vi "Headless Video Analyzer.vi"() -> ()   [LabVIEW 2018]
uses:
  Shared/Roughness Parameters STYP.ctl
  Classes/Message/Message.lvclass
  Private/Headless Video Analyzer Status STYP.ctl
  Classes/Video File/Video File.lvclass
  Classes/Video Frame/Video Frame.lvclass
  <vilib>/vision/Image Controls.llb/IMAQ Image.ctl
  <userlib>/Jet Engineering/JET_QSM/Code/Private/JET_QSM_InvalidOption STYP.ctl
  Classes/Video File/Video File.lvclass/Video File.ctl
  <userlib>/Jet Engineering/JET_QSM/Code/Private/JET_QSM - Add State [String API].vi
  905395b3-fc2a-4912-8404-34f757d12cd7.vi
  Classes/Video File/Read Number of Frames.vi
  Classes/Video File/Read Frame Number.vi
  Datalogger/Messages/Datalogger Headers Set Message/Datalogger Headers Set Message.lvclass
  C:/Users/aaron.jencks/Documents/GitHub/emerson_seed_object_detection/LabVIEW/Projects/Paul's Video Viewer/Classes/Message/Message.lvclass
  Datalogger/Messages/Datalogger Data Save Message.lvclass
  Classes/STOP Message/STOP.lvclass
  Classes/Depth Data Message/Depth Data Message.lvclass
  <vilib>/Utility/error.llb/Trim Whitespace.vi
  <vilib>/Utility/error.llb/Error Cluster From Error Code.vi
panel:
  out "Frame Number":u32
  out "Progress":dbl(slide) scale=0.0..100.0
  out "Depth":T1(plugin-control)
  out "Ready?":bool
  in  "stop":bool
  out "File Opened?":bool
  out "Frame Count":u32
  out "Roughness Parameters":T2
  in  "Path":path
  out "RGB":T1(plugin-control)
  out "Recent states before Error (with tick counts) 2":string="0.167 sec ago: VI Initialize\n0.167 sec ago: Window Open\n0.110 sec ago: Control Update\n0.110 sec ago: Indicator Update\n0.000 sec ago: Error Handler\r\n"
  out "error out":errorcluster
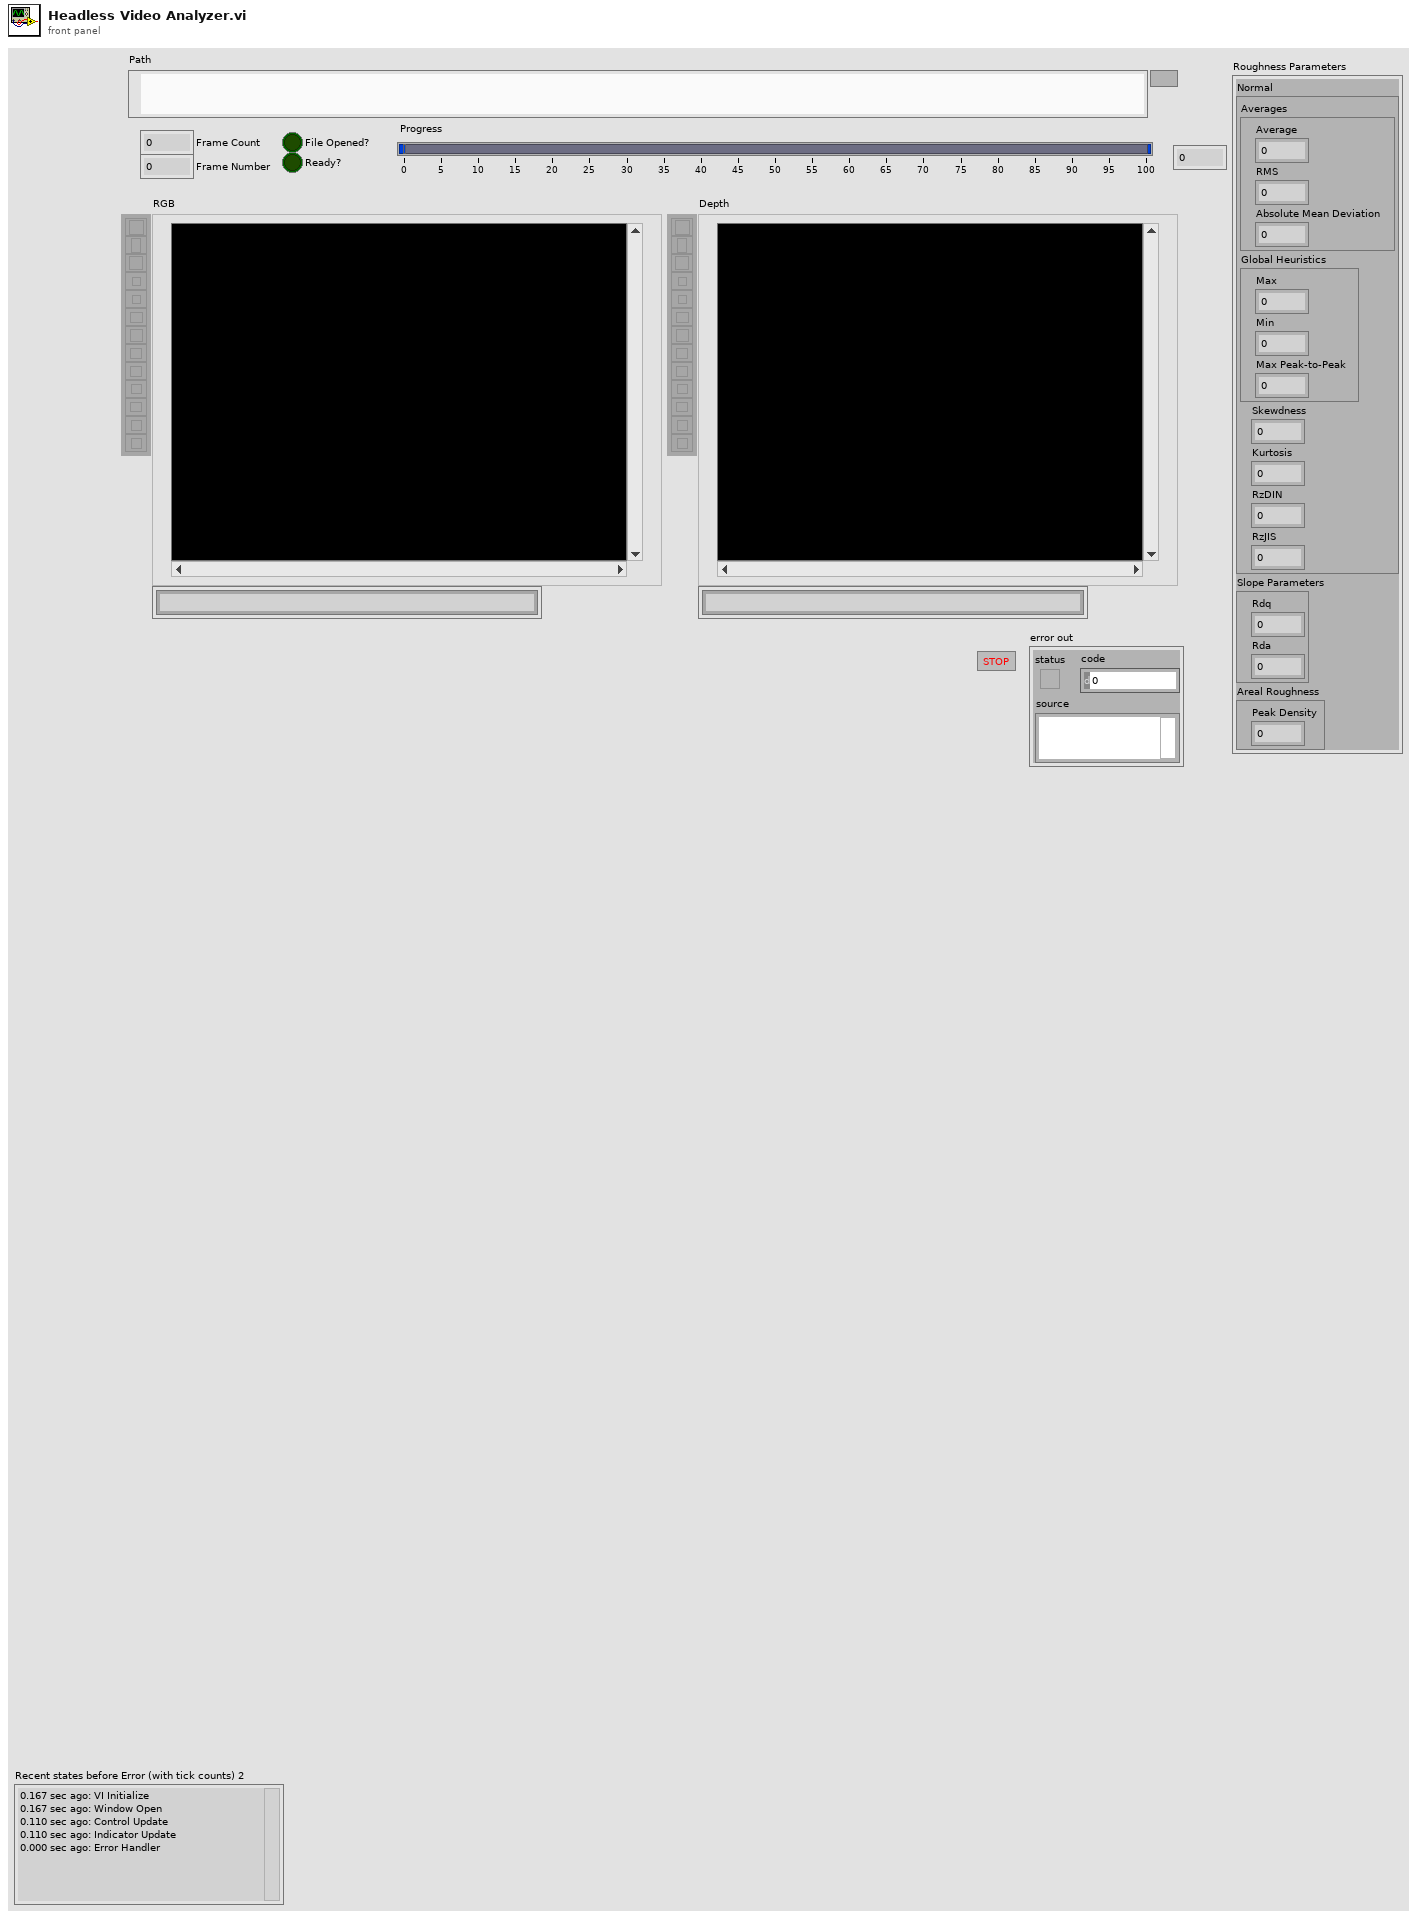
[diagram p1: front panel]
types:
  T1 = typedef "IMAQ Image.ctl" = refnum<image>
  T2 = typedef "Roughness Parameters STYP.ctl" = cluster{"Normal":cluster{"Averages":cluster{"Average":dbl, "RMS":dbl, "Absolute Mean Deviation":dbl}, "Global Heuristics":cluster{"Max":dbl, "Min":dbl, "Max Peak-to-Peak":dbl}, "Skewdness":dbl, "Kurtosis":dbl, "RzDIN":dbl, "RzJIS":dbl}, "Slope Parameters":cluster{"Rdq":dbl, "Rda":dbl}, "Areal Roughness":cluster{"Peak Density":dbl}}
  T3 = typedef "Headless Video Analyzer Status STYP.ctl" = cluster{"VI":cluster{"error":errorcluster, "isExiting?":bool}, "UserLoggedIn?":bool, "data log queue":refnum<queue>, "stop queue":refnum<queue>, "ready queue":refnum<queue>, "Files":cluster{"Depth File":refnum<class "Video File.lvclass">, "RGB File":refnum<class "Video File.lvclass">}, "Frames":cluster{"Depth Frame":refnum<class "Video Frame.lvclass">, "RGB Frame":refnum<class "Video Frame.lvclass">}, "Images":cluster{"Depth Placeholder":T1, "RGB Placeholder":T1}, "Playing?":bool, "Processed Frame":T2}
  T4 = typedef "JET_QSM_InvalidOption STYP.ctl" = enum16{"Ignore", "Dialog", "Error"}
  T5 = typedef "JET_QSM_Refnum STYP.ctl" = cluster{"state":cluster{"queue":refnum<queue>, "idle":string, "error":string, "STOP":string}, "debug":cluster{"enabled?":bool, "queue":refnum<queue>}, "Invalid.option":T4, "QSM.Name":string}
  T6 = enum32{"invalid app kind", "Development System", "Run Time System", "Student Edition", "Embedded LabVIEW", "Evaluation", "Custom"}
  T7 = typedef "JET_QSM_Element STYP.ctl" = cluster{"state":string, "data":variant, "comment":string}
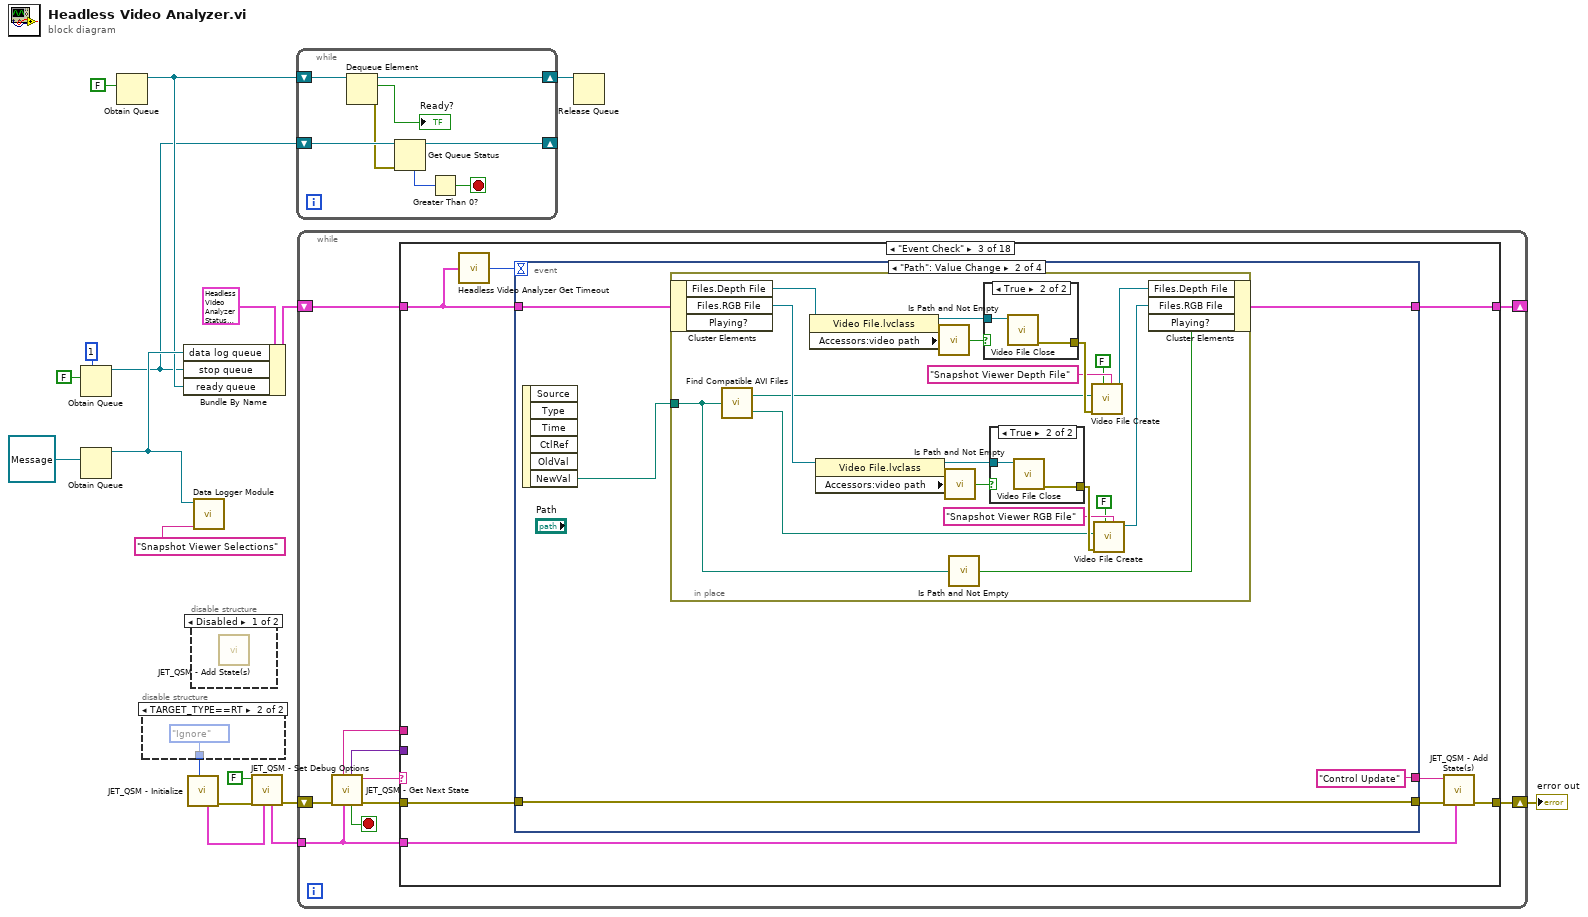
[diagram p0: block diagram]
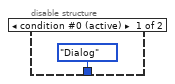
[diagram p2: hidden frame]
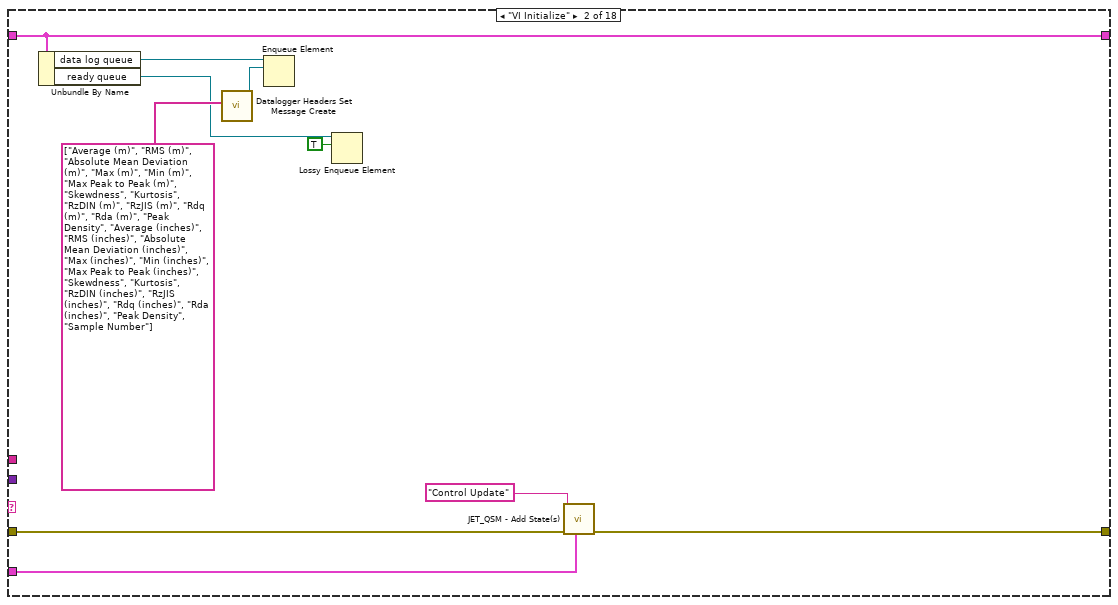
[diagram p5: hidden frame]
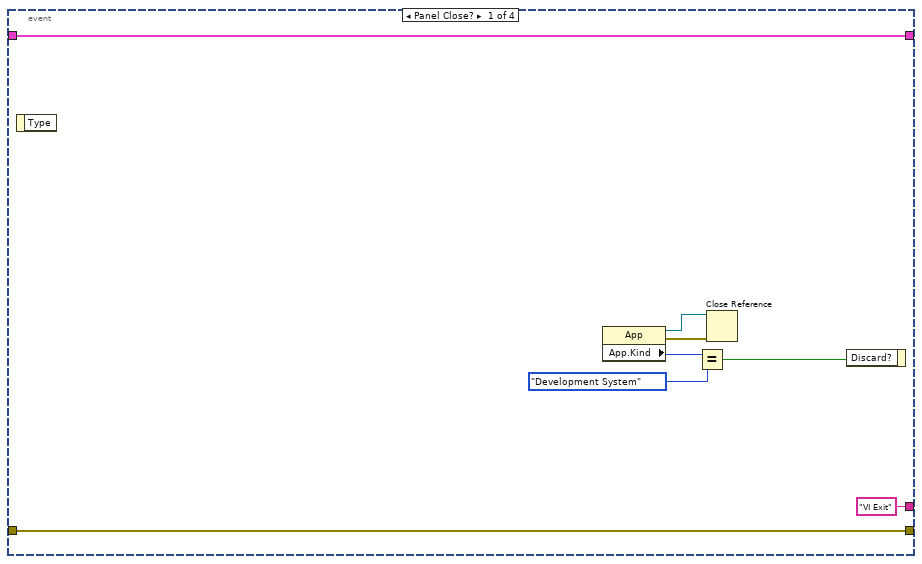
[diagram p6: hidden frame]
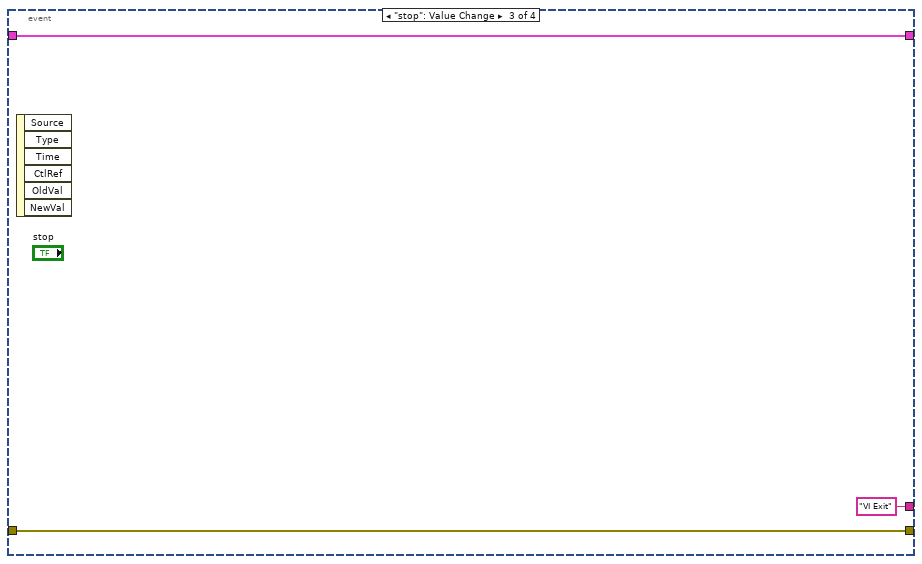
[diagram p9: hidden frame]
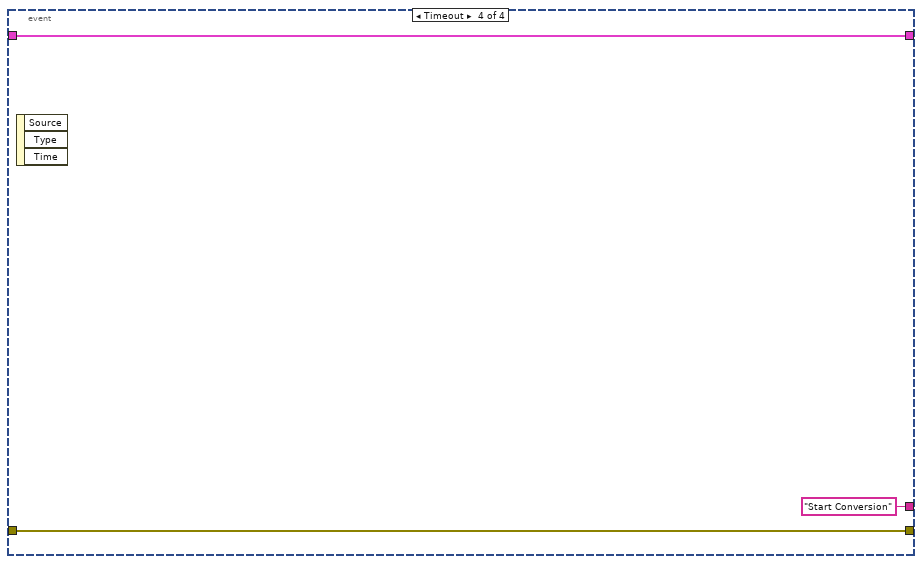
[diagram p10: hidden frame]
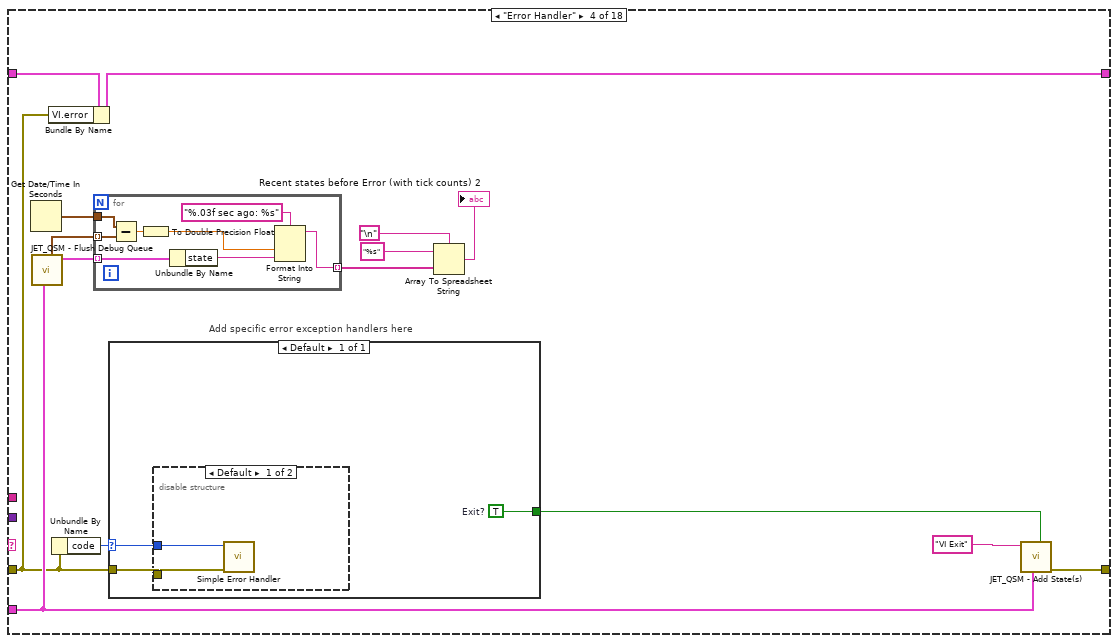
[diagram p11: hidden frame]
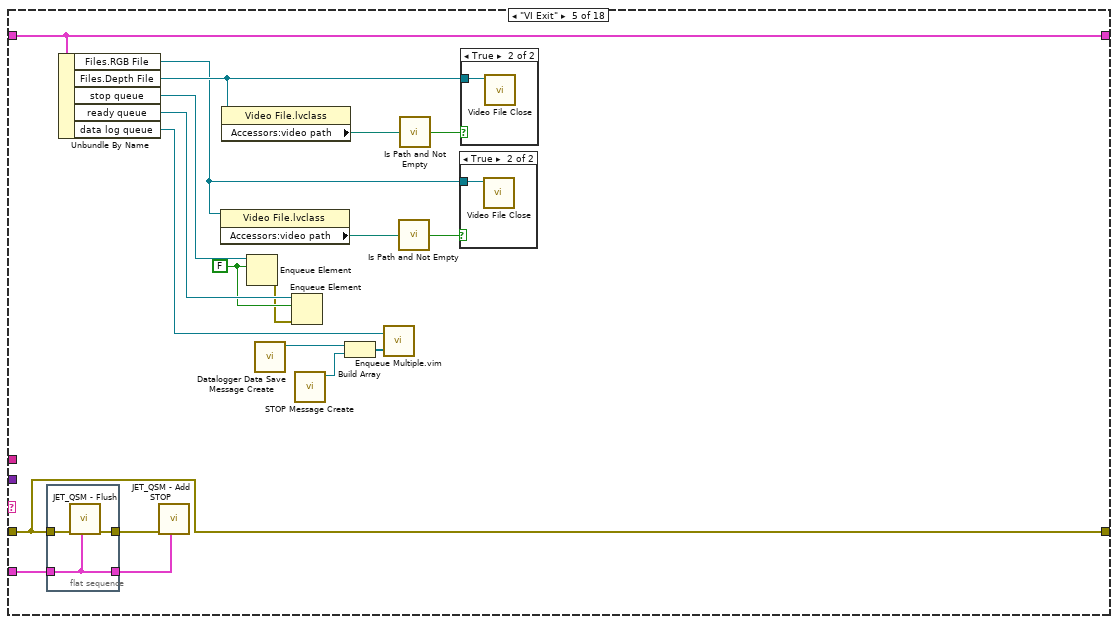
[diagram p13: hidden frame]
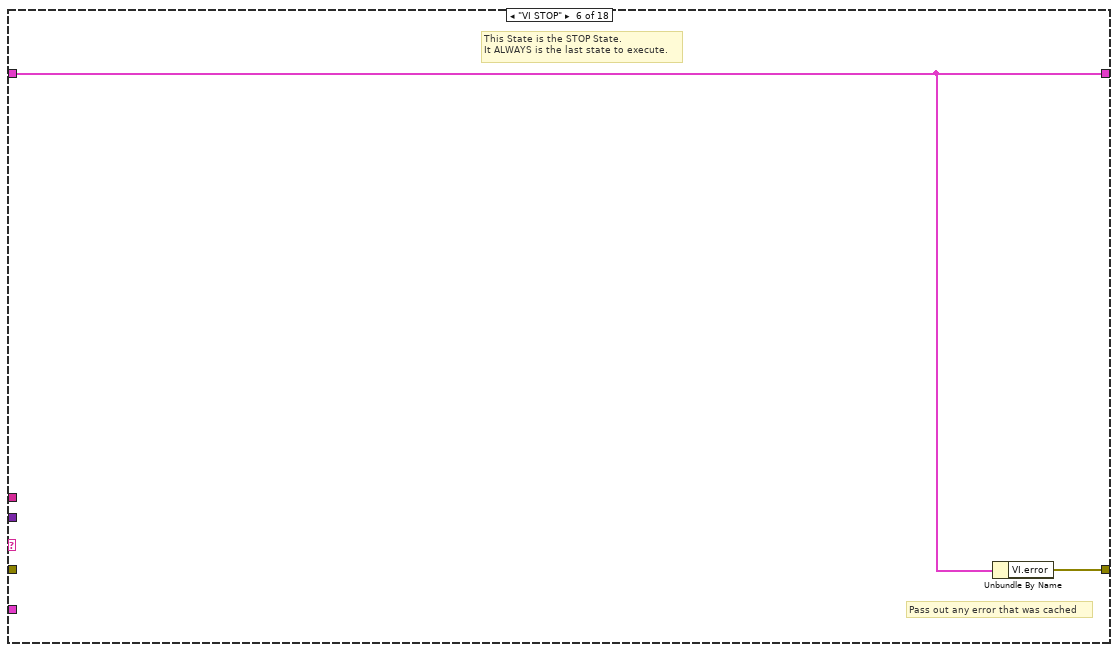
[diagram p16: hidden frame]
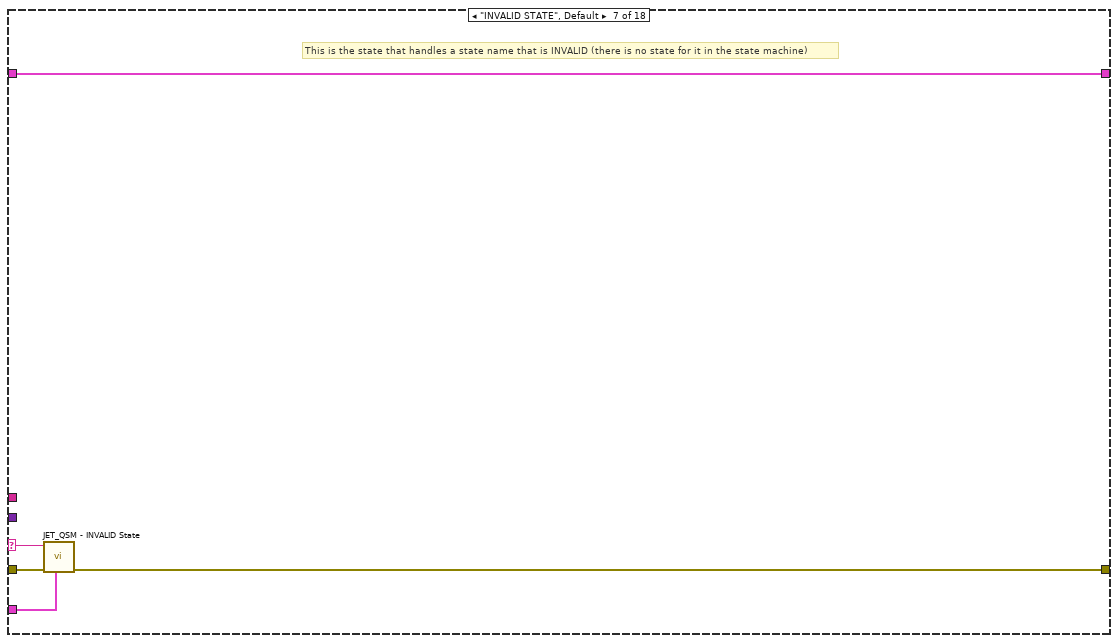
[diagram p17: hidden frame]
diagram:
  n1 = Obtain Queue(max queue size (-1, unlimited)=1, element data type=FALSE) -> (queue out=w4:refnum<queue>)  [unwired: 3 in, 2 out]
  n2 = Obtain Queue(element data type=refnum<class "Message.lvclass"> refnum ("Message.lvclass")) -> (queue out=w8:refnum<queue>)  [unwired: 4 in, 2 out]
  n3 = Obtain Queue(element data type=FALSE) -> (queue out=w5:refnum<queue>)  [unwired: 4 in, 2 out]
  n4 = disable-structure shown="TARGET_TYPE==RT" {
    disable-tunnel: [JET_QSM_InvalidOption_STYP."Dialog" ("invalid state action (Dialog)") JET_QSM_InvalidOption_STYP."Ignore" ("invalid state action (Dialog)")] -> w18
    frame condition #0 (active) {
    }
    frame condition #1 {
    }
  }
  n5 = Bundle By Name(cluster=T3 {"VI"={"error"={"status"=FALSE, "code"=0, "source"=""}, "isExiting?"=FALSE}, "UserLoggedIn?"=FALSE, "data log queue"=refnum, "stop queue"=refnum, "ready queue"=refnum, "Files"={"Depth File"=refnum, "RGB File"=refnum}, "Frames"={"Depth Frame"=refnum, "RGB Frame"=refnum}, "Images"={"Depth Placeholder"=refnum, "RGB Placeholder"=refnum}, "Playing?"=FALSE, "Processed Frame"={"Normal"={"Averages"={"Average"=0.0, "RMS"=0.0, "Absolute Mean Deviation"=0.0}, "Global Heuristics"={"Max"=0.0, "Min"=0.0, "Max Peak-to-Peak"=0.0}, "Skewdness"=0.0, "Kurtosis"=0.0, "RzDIN"=0.0, "RzJIS"=0.0}, "Slope Parameters"={"Rdq"=0.0, "Rda"=0.0}, "Areal Roughness"={"Peak Density"=0.0}}} ("Status"), "data log queue"=w8, "stop queue"=w4, "ready queue"=w5) -> (w9:T3)
  n6 = call <userlib>:"JET_QSM - Initialize.vi"("invalid state action (Dialog)"=w18) -> ("error out"=w12:errorcluster, "Jet_QSM refnum"=w15:T5)  [unwired: 9 in]
  n7 = disable-structure shown="Disabled" {
    frame Disabled {
      n8 = call-poly <userlib>:"JET_QSM - Add State(s).vi"() -> ()  [unwired: 11 in, 1 out]
    }
    frame Enabled {
    }
  }
  n9 = call "Data Logger Module.vi"("Identifier"="Snapshot Viewer Selections", "Message queue"=w8) -> ()  [unwired: 10 in]
  n10 = call <userlib>:"JET_QSM - Set Debug Options.vi"("Jet_QSM refnum"=w15, "error in (no error)"=w12, "debug.enabled? (F)"=FALSE) -> ("error out"=w13:errorcluster, "Jet_QSM ref"=w14:T5)  [unwired: 7 in]
  n11 = while {
    shift-right: [w26] -> w3
    shift-left: w5 -> [w28]
    shift-right: [w22] -> _
    shift-left: w4 -> [w25]
    stop <- w23 stop-if-true
    n12 = Dequeue Element(queue=w28) -> (queue out=w26:refnum<queue>, element=→"Ready?":bool, error out=w21:errorcluster)  [unwired: 2 in, 1 out]
    n13 = Get Queue Status(queue=w25, error in (no error)=w21) -> (queue out=w22:refnum<queue>, # elements in queue=w24:i32)  [unwired: 1 in, 6 out]
    n14 = Greater Than 0?(x=w24) -> (x > 0?=w23:bool)
  }
  n15 = while {
    tunnel: w14 -> [w34]
    shift-right: [w32] -> _
    shift-left: w9 -> [w33]
    shift-right: [w31] -> w17
    shift-left: w13 -> [w38]
    stop <- w35 stop-if-true
    n16 = call <userlib>:"JET_QSM - Get Next State.vi"("Jet_QSM refnum"=w34, "error in (no error)"=w38) -> ("error out"=w37:errorcluster, "state"=w36:string, "Stop Loop?"=w35:bool, "state data"=w30:variant, "state comment"=w29:string)  [unwired: 5 in]
    n17 = case shown="\"Event Check\"" w36 {
      selector: w36 -> [_ _ _ _ _ _ w158 _ _ _ _ _ _ _ _ _ _ _]
      tunnel: w37 -> [w39 w49 w58 w103 w148 _ w159 w161 w163 w165 w174 w193 w210 w215 w219 w220 w226 w246]
      tunnel: w34 -> [_ w50 w57 w108 w146 _ w157 _ _ _ w172 _ _ _ _ _ w227 _]
      tunnel: w33 -> [w40 w46 w52 w104 w144 w154 w160 w162 w164 w166 w170 w192 w208 w211 w218 w221 w224 w245]
      tunnel: [w40 w46 w53 w102 w144 w154 w160 w162 w164 w166 w170 w190 w206 w211 w218 w221 w224 w245] -> w32
      tunnel: [w39 w48 w55 w109 w148 w155 w156 w161 w163 w165 w173 w193 w210 w215 w219 w220 w225 w246] -> w31
      tunnel: w30 -> [_ _ _ _ _ _ _ _ _ _ _ _ _ _ _ _ _ _]
      tunnel: w29 -> [_ _ _ _ _ _ _ _ _ _ _ _ _ _ _ _ _ _]
      frame "------ Standard States ------" {
        # "Standard States are required states for a JET_QSM State Machine\n\nTheir names may be changed; use the Initialize function to specify the new names"
        # "This is a section header; the state is never expected to execute"
      }
      frame "VI Initialize" {
        n18 = Unbundle By Name(w46) -> ("data log queue"=w45:refnum<queue>, "ready queue"=w42:refnum<queue>)
        n19 = call "Datalogger Headers Set Message Create.vi"("Headers"=string[] ["Average (m)", "RMS (m)", "Absolute Mean Deviation (m)", "Max (m)", "Min (m)", "Max Peak to Peak (m)", "Skewdness", "Kurtosis", "RzDIN (m)", "RzJIS (m)", "Rdq (m)", "Rda (m)", "Peak Density", "Average (inches)", "RMS (inches)", "Absolute Mean Deviation (inches)", "Max (inches)", "Min (inches)", "Max Peak to Peak (inches)", "Skewdness", "Kurtosis", "RzDIN (inches)", "RzJIS (inches)", "Rdq (inches)", "Rda (inches)", "Peak Density", "Sample Number"]) -> ("Datalogger Headers Set Message out"=w44:refnum<class "Datalogger Headers Set Message.lvclass">)  [unwired: 9 in, 1 out]
        n20 = Enqueue Element(queue=w45, element=w44) -> ()  [unwired: 2 in, 3 out]
        n21 = Lossy Enqueue Element(queue=w42, element=TRUE) -> ()  [unwired: 1 in, 4 out]
        n22 = call-poly <userlib>:"JET_QSM - Add State(s).vi"("Jet_QSM refnum"=w50, "error in (no error)"=w49, "state(s)"="Control Update") -> ("error out"=w48:errorcluster)  [unwired: 8 in]
      }
      frame "Event Check" {
        n23 = call "Headless Video Analyzer Get Timeout.vi"("Status"=w52) -> ("timeout"=w51:i32)
        n24 = event shown="[1] \"Path\": Value Change" {
          selector: _ -> [_ _ _ _]
          dyn-events: _ -> [_ _ _ _]
          timeout: w51 -> [_ _ _ _]
          tunnel: w58 -> [w60 w71 w97 w100]
          tunnel: ["VI Exit" ("state(s)") "Control Update" ("state(s)") "VI Exit" ("state(s)") "Start Conversion" ("state(s)")] -> w56
          tunnel: [w60 w71 w97 w100] -> w54
          tunnel: w52 -> [w59 w69 w98 w101]
          tunnel: [w59 w68 w98 w101] -> w53
          event Panel Close? {
            n25 = event-data() -> ()  [unwired: 1 in, 1 out]
            n26 = property class="App"() -> (reference out=w62:refnum<vi>, error out=w63:errorcluster, "App.Kind"=w66:T6)  [unwired: 2 in]
            n27 = Equal?(x=w66, y=T6."Development System") -> (x = y?=w64:bool)
            n28 = Close Reference(reference=w62, error in (no error)=w63) -> ()  [unwired: 1 out]
            n29 = event-data("Discard?"=w64) -> ()  [unwired: 1 in, 1 out]
          }
          event "Path": Value Change {
            n30 = event-data() -> ("NewVal"=w67:path)  [unwired: 1 in, 5 out]
            n31 = in-place {
              in-place-border: w67 -> [w75]
              n32 = in-place-cluster #1(w69) -> ("Files.Depth File"=w91:refnum<class "Video File.lvclass">, "Files.RGB File"=w84:refnum<class "Video File.lvclass">)  [unwired: 1 out]
              n33 = call "Find Compatible AVI Files.vi"("Video Path"=w75) -> ("RGB Path"=w76:path, "Depth Path"=w77:path)  [unwired: 2 in]
              n34 = property class="Video File.lvclass"(reference=w91) -> (reference out=w88:refnum<class "Video File.lvclass">, "Accessors:video path"=w90:path)  [unwired: 1 in, 1 out]
              n35 = property class="Video File.lvclass"(reference=w84) -> (reference out=w82:refnum<class "Video File.lvclass">, "Accessors:video path"=w83:path)  [unwired: 1 in, 1 out]
              n36 = call <vilib>:"Is Path and Not Empty.vi"("path"=w90) -> ("Is Path and Not Empty?"=w89:bool)  [unwired: 4 in]
              n37 = call <vilib>:"Is Path and Not Empty.vi"("path"=w83) -> ("Is Path and Not Empty?"=w81:bool)  [unwired: 4 in]
              n38 = call <vilib>:"Is Path and Not Empty.vi"("path"=w75) -> ("Is Path and Not Empty?"=w74:bool)  [unwired: 4 in]
              n39 = case shown="True" w89 {
                tunnel: w88 -> [_ w95]
                tunnel: [_ w94] -> w86
                frame False {
                }
                frame True {
                  n40 = call-dynamic "Video File Close.vi"("Video File in"=w95) -> ("error out"=w94:errorcluster)  [unwired: 9 in, 1 out]
                }
              }
              n41 = case shown="True" w81 {
                tunnel: w82 -> [_ w93]
                tunnel: [_ w92] -> w80
                frame False {
                }
                frame True {
                  n42 = call-dynamic "Video File Close.vi"("Video File in"=w93) -> ("error out"=w92:errorcluster)  [unwired: 9 in, 1 out]
                }
              }
              n43 = call "Video File Create.vi"("Identifier"="Snapshot Viewer Depth File", "Loop? (T)"=FALSE, "error in (no error)"=w86, "Video Path (\"\")"=w77) -> ("Video File out"=w87:refnum<class "Video File.lvclass">)  [unwired: 6 in, 1 out]
              n44 = call "Video File Create.vi"("Identifier"="Snapshot Viewer RGB File", "Loop? (T)"=FALSE, "error in (no error)"=w80, "Video Path (\"\")"=w76) -> ("Video File out"=w78:refnum<class "Video File.lvclass">)  [unwired: 6 in, 1 out]
              n45 = in-place-cluster #1("Files.Depth File"=w87, "Files.RGB File"=w78, "Playing?"=w74) -> (w68:T3)
            }
          }
          event "stop": Value Change {
            n46 = event-data() -> ()  [unwired: 1 in, 6 out]
          }
          event Timeout {
            n47 = event-data() -> ()  [unwired: 1 in, 3 out]
          }
        }
        n48 = call-poly <userlib>:"JET_QSM - Add State(s).vi"("Jet_QSM refnum"=w57, "error in (no error)"=w54, "state(s)"=w56) -> ("error out"=w55:errorcluster)  [unwired: 8 in]
      }
      frame "Error Handler" {
        # "Add specific error exception handlers here"
        n49 = Get Date/Time In Seconds() -> (seconds since 1Jan1904=w112:timestamp)
        n50 = call <userlib>:"JET_QSM - Flush Debug Queue.vi"("Jet_QSM refnum"=w108) -> ("QSM Elements"=w110:T7[], "Timestamps"=w111:timestamp[])  [unwired: 8 in, 1 out]
        n51 = Bundle By Name(cluster=w104, "VI.error"=w103) -> (w102:T3)
        n52 = Unbundle By Name(w103) -> ("code"=w105:i32)
        n53 = for {
          tunnel: w110 -> [w124] mode=indexing
          tunnel: [w122] -> w114 mode=indexing
          tunnel: w112 -> [w119]
          tunnel: w111 -> [w120] mode=indexing
          n54 = Subtract(x=w119, y=w120) -> (x-y=w118:dbl)
          n55 = To Double Precision Float(number=w118) -> (double precision float=w117:dbl)
          n56 = Unbundle By Name(w124) -> ("state"=w123:string)
          n57 = Format Into String(format string="%.03f sec ago: %s", w117, w123) -> (resulting string=w122:string)  [unwired: 2 in, 1 out]
        }
        n58 = case shown="Default" w105 {
          selector: w105 -> [w126]
          tunnel: [w127] -> w106
          tunnel: w103 -> [w125]
          frame Default {
            w127 = TRUE  # Exit?
            n59 = disable-structure shown="Default" {
              disable-tunnel: w126 -> [w129 _]
              disable-tunnel: w125 -> [w128 _]
              frame condition #0 (active) {
                n60 = call <vilib>:"Simple Error Handler.vi"("error code (no error:0)"=w129, "error in (no error)"=w128) -> ()  [unwired: 3 in, 5 out]
              }
              frame condition #1 {
              }
            }
          }
        }
        n61 = Array To Spreadsheet String(delimiter (Tab)="\n", array=w114, 3:"%s" ("format string")) -> (spreadsheet string=→"Recent states before Error (with tick counts) 2":string)
        n62 = call-poly <userlib>:"JET_QSM - Add State(s).vi"("act? (T)"=w106, "Jet_QSM refnum"=w108, "state(s)"="VI Exit") -> ("error out"=w109:errorcluster)  [unwired: 8 in]
      }
      frame "VI Exit" {
        w138 = FALSE ("element")
        n63 = flat-sequence {
          tunnel: w148 -> [w153]
          tunnel: [w152] -> w147
          tunnel: w146 -> [w151]
          tunnel: [w151] -> w145
          frame #0 {
            n64 = call <userlib>:"JET_QSM - Flush.vi"("Jet_QSM ref"=w151, "error in (no error)"=w153) -> ("error out"=w152:errorcluster)  [unwired: 8 in, 1 out]
          }
        }
        n65 = Unbundle By Name(w144) -> ("Files.RGB File"=w130:refnum<class "Video File.lvclass">, "Files.Depth File"=w141:refnum<class "Video File.lvclass">, "stop queue"=w140:refnum<queue>, "ready queue"=w139:refnum<queue>, "data log queue"=w134:refnum<queue>)
        n66 = call <userlib>:"JET_QSM - Add STOP.vi"("Jet_QSM refnum"=w145, "error in (no error)"=w147) -> ()  [unwired: 9 in, 1 out]
        n67 = property class="Video File.lvclass"(reference=w130) -> ("Accessors:video path"=w132:path)  [unwired: 1 in, 2 out]
        n68 = property class="Video File.lvclass"(reference=w141) -> ("Accessors:video path"=w143:path)  [unwired: 1 in, 2 out]
        n69 = Enqueue Element(queue=w140, element=w138) -> (error out=w137:errorcluster)  [unwired: 2 in, 2 out]
        n70 = call "Datalogger Data Save Message Create.vi"() -> ("Datalogger Data Save Message out"=w136:refnum<class "Datalogger Data Save Message.lvclass">)  [unwired: 10 in, 1 out]
        n71 = Enqueue Element(queue=w139, element=w138, error in (no error)=w137) -> ()  [unwired: 1 in, 3 out]
        n72 = call "STOP Message Create.vi"() -> ("STOP out"=w135:refnum<class "STOP.lvclass">)  [unwired: 10 in, 1 out]
        n73 = Build Array(w136, w135) -> (w133:refnum<class "Message.lvclass">[])
        n74 = call "Enqueue Multiple.vim"("Array"=w133, "queue out"=w134) -> ()  [unwired: 1 out]
        n75 = call <vilib>:"Is Path and Not Empty.vi"("path"=w132) -> ("Is Path and Not Empty?"=w131:bool)  [unwired: 4 in]
        n76 = call <vilib>:"Is Path and Not Empty.vi"("path"=w143) -> ("Is Path and Not Empty?"=w142:bool)  [unwired: 4 in]
        n77 = case shown="True" w131 {
          tunnel: w130 -> [_ w149]
          frame False {
          }
          frame True {
            n78 = call-dynamic "Video File Close.vi"("Video File in"=w149) -> ()  [unwired: 9 in, 2 out]
          }
        }
        n79 = case shown="True" w142 {
          tunnel: w141 -> [_ w150]
          frame False {
          }
          frame True {
            n80 = call-dynamic "Video File Close.vi"("Video File in"=w150) -> ()  [unwired: 9 in, 2 out]
          }
        }
      }
      frame "VI STOP" {
        # "Pass out any error that was cached"
        # "This State is the STOP State.\nIt ALWAYS is the last state to execute."
        n81 = Unbundle By Name(w154) -> ("VI.error"=w155:errorcluster)
      }
      frame "INVALID STATE", Default {
        # "This is the state that handles a state name that is INVALID (there is no state for it in the state machine)"
        n82 = call <userlib>:"JET_QSM - INVALID State.vi"("Jet_QSM refnum"=w157, "error in (no error)"=w159, "state"=w158) -> ("error out"=w156:errorcluster)  [unwired: 8 in]
      }
      frame "------ Menu Commands ------" {
        # "This is a section header; the state is never expected to execute"
      }
      frame "------ Events  ------" {
        # "This is a section header; the state is never expected to execute"
      }
      frame "------ Actions  ------" {
        # "This is a section header; the state is never expected to execute"
      }
      frame "Start Conversion" {
        n83 = Unbundle By Name(w170) -> ("ready queue"=w169:refnum<queue>, "Playing?"=w167:bool)
        n84 = call-poly <userlib>:"JET_QSM - Add State(s).vi"("act? (T)"=w167, "Jet_QSM refnum"=w172, "error in (no error)"=w174, "state(s)"="Read Frame\nProcess Frame\nLog Data\nControl Update") -> ("error out"=w173:errorcluster)  [unwired: 7 in]
        n85 = Not(x=w167) -> (.not. x?=w168:bool)
        n86 = Lossy Enqueue Element(queue=w169, element=w168) -> ()  [unwired: 1 in, 4 out]
      }
      frame "Read Frame" {
        n87 = Unbundle By Name(w192) -> ("Files.RGB File"=w187:refnum<class "Video File.lvclass">, "Files.Depth File"=w183:refnum<class "Video File.lvclass">, "Images.Depth Placeholder"=w180:T1, "Images.RGB Placeholder"=w179:T1)
        n88 = property class="Video File.lvclass"(reference=w183) -> (reference out=w189:refnum<class "Video File.lvclass">, "Accessors:video path"=w182:path)  [unwired: 1 in, 1 out]
        n89 = property class="Video File.lvclass"(reference=w187) -> (reference out=w186:refnum<class "Video File.lvclass">, "Accessors:video path"=w181:path)  [unwired: 1 in, 1 out]
        n90 = call <vilib>:"Is Path and Not Empty.vi"("path"=w181) -> ("Is Path and Not Empty?"=w185:bool)  [unwired: 4 in]
        n91 = call <vilib>:"Is Path and Not Empty.vi"("path"=w182) -> ("Is Path and Not Empty?"=w188:bool)  [unwired: 4 in]
        n92 = case shown="False" w188 {
          tunnel: [_ w204] -> w191
          tunnel: w189 -> [w199 w203]
          tunnel: w180 -> [_ w202]
          tunnel: [_ w201] -> w178
          tunnel: [w199 w200] -> w176
          frame False {
          }
          frame True {
            n93 = call-dynamic "Video File Frame Read.vi"("Image Dst"=w202, "Video File in"=w203) -> ("Video Frame out"=w204:refnum<class "Video Frame.lvclass">, "Video File out"=w200:refnum<class "Video File.lvclass">, "Playback Finished?"=w201:bool)  [unwired: 5 in, 2 out]
          }
        }
        n94 = case shown="False" w185 {
          tunnel: w179 -> [_ w198]
          tunnel: [_ w197] -> w184
          tunnel: w186 -> [w194 w196]
          tunnel: [w194 w195] -> w175
          frame False {
          }
          frame True {
            n95 = call-dynamic "Video File Frame Read.vi"("Image Dst"=w198, "Video File in"=w196) -> ("Video Frame out"=w197:refnum<class "Video Frame.lvclass">, "Video File out"=w195:refnum<class "Video File.lvclass">)  [unwired: 5 in, 3 out]
          }
        }
        n96 = Not(x=w178) -> (.not. x?=w177:bool)
        n97 = Bundle By Name(cluster=w192, "Files.Depth File"=w176, "Files.RGB File"=w175, "Frames.Depth Frame"=w191, "Frames.RGB Frame"=w184, "Playing?"=w177) -> (w190:T3)
      }
      frame "Process Frame" {
        n98 = Unbundle By Name(w208) -> ("Frames.Depth Frame"=w209:refnum<class "Video Frame.lvclass">)
        n99 = call "Compute Roughness Params.vi"("Video Frame"=w209, "Full? (T)"=TRUE) -> ("Roughness Parameters"=w207:T2)  [unwired: 3 in]
        n100 = Bundle By Name(cluster=w208, "Processed Frame"=w207) -> (w206:T3)
      }
      frame "Log Data" {
        n101 = Unbundle By Name(w211) -> ("Processed Frame"=w213:T2, "data log queue"=w212:refnum<queue>)
        n102 = call "Depth Data Message Create.vi"("Roughness"=w213) -> ("Depth Data Message out"=w214:refnum<class "Depth Data Message.lvclass">)  [unwired: 9 in, 1 out]
        n103 = Enqueue Element(queue=w212, element=w214) -> ()  [unwired: 2 in, 3 out]
      }
      frame "Log Save" {
        n104 = Unbundle By Name(w218) -> ("data log queue"=w217:refnum<queue>)
        n105 = call "Datalogger Data Save Message Create.vi"() -> ("Datalogger Data Save Message out"=w216:refnum<class "Datalogger Data Save Message.lvclass">)  [unwired: 10 in, 1 out]
        n106 = Enqueue Element(queue=w217, element=w216) -> ()  [unwired: 2 in, 3 out]
      }
      frame "------ Window and Panel Control ------" {
        # "This is a section header; the state is never expected to execute"
      }
      frame "Control Update" {
        # "Update all control properties here from the status cluster\n(Consolidate/reduce property nodes)"
        n107 = Unbundle By Name(w224) -> ("Files.Depth File"=w223:refnum<class "Video File.lvclass">)
        n108 = property class="Video File.lvclass"(reference=w223) -> ("Accessors:video path"=w222:path)  [unwired: 1 in, 2 out]
        n109 = local write "Path"(w222) -> ()
        n110 = call-poly <userlib>:"JET_QSM - Add State(s).vi"("Jet_QSM refnum"=w227, "error in (no error)"=w226, "state(s)"="Indicator Update") -> ("error out"=w225:errorcluster)  [unwired: 8 in]
      }
      frame "Indicator Update" {
        # "Update all indicator values here from the status cluster\n(Eliminate Local Variables)"
        n111 = Unbundle By Name(w245) -> ("Files.Depth File"=w244:refnum<class "Video File.lvclass">, "Frames.Depth Frame"=w242:refnum<class "Video Frame.lvclass">, "Frames.RGB Frame"=w230:refnum<class "Video Frame.lvclass">, "Processed Frame"=→"Roughness Parameters":T2)
        n112 = property class="Video Frame.lvclass"(reference=w230) -> ("Accessors:Image"=→"RGB":T1)  [unwired: 1 in, 2 out]
        n113 = property class="Video Frame.lvclass"(reference=w242) -> ("Accessors:Image"=→"Depth":T1)  [unwired: 1 in, 2 out]
        n114 = property class="Video File.lvclass"(reference=w244) -> ("Accessors:video path"=w243:path, "Accessors:Number of Frames"=w238:u32, "Accessors:Frame Number"=w237:u32)  [unwired: 1 in, 2 out]
        "Frame Count" <- w238
        "Frame Number" <- w237
        n115 = call <vilib>:"Is Path and Not Empty.vi"("path"=w243) -> ("Is Path and Not Empty?"=→"File Opened?":bool)  [unwired: 4 in]
        n116 = Increment(x=w237) -> (x+1=w231:u32)
        n117 = To Double Precision Float(number=w238) -> (double precision float=w235:dbl)
        n118 = To Double Precision Float(number=w231) -> (double precision float=w236:dbl)
        n119 = Divide(x=w236, y=w235) -> (x/y=w234:dbl)
        n120 = Multiply(x=100.0, y=w234) -> (x*y=→"Progress":dbl)
      }
    }
  }
  "error out" <- w17
  n121 = Release Queue(queue=w3) -> ()  [unwired: 2 in, 3 out]
